vi "Set Is From Actor.vi"(10 "Is From Actor":bool, 11 "Base Sender in":refnum<class "Base Sender.lvclass">) -> (3 "Base Sender out":refnum<class "Base Sender.lvclass">)   [LabVIEW 2020, in "jettl.lvlib" / "Sender.lvlib" / "Base Sender.lvclass"]
uses:
  Base Sender.lvclass
  Base Sender.lvclass/Base Sender.ctl
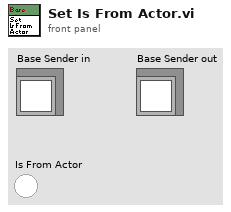
[diagram p1: front panel]
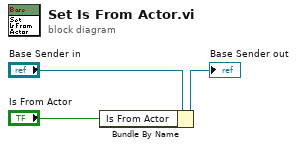
[diagram p0: block diagram]
diagram:
  n1 = Bundle By Name(cluster="Base Sender in", "Is From Actor"="Is From Actor") -> (→"Base Sender out":refnum<class "Base Sender.lvclass">)
